vi "GetTunnels.vi"(6 "error in":errorcluster, 9 "CaseStructure in":refnum<class "CaseStructure.lvclass">) -> (0 "error out":errorcluster, 3 "CaseStructure out":refnum<class "CaseStructure.lvclass">, 4 "Tunnels":i32[](array[numeric]))   [LabVIEW 2014, in "CaseStructure.lvclass"]
uses:
  CaseStructure.lvclass
  Structure/Structure.lvclass
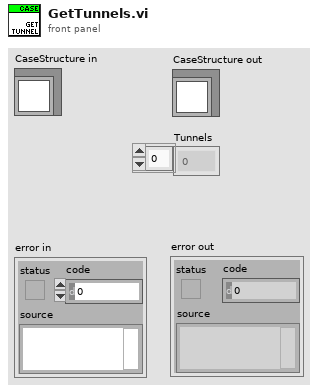
[diagram p1: front panel]
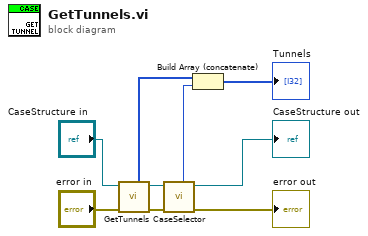
[diagram p0: block diagram]
diagram:
  n1 = call-parent "GetTunnels.vi"("error in"="error in", "Structure in"="CaseStructure in") -> ("error out"=w5:errorcluster, "Structure out"=w6:refnum<class "CaseStructure.lvclass">, "Tunnels"=w9:i32[])  [unwired: 5 in]
  n2 = call "CaseSelector.vi"("error in"=w5, "CaseStructure in"=w6) -> ("error out"=→"error out":errorcluster, "CaseStructure out"=→"CaseStructure out":refnum<class "CaseStructure.lvclass">, "Selector.UID"=w1:i32)  [unwired: 5 in]
  n3 = Build Array (concatenate)(w9, w1) -> (→"Tunnels":i32[])
